vi "SVFA Zoom FFT Spectrum (Mag-Phase).vi"   [LabVIEW 2017]
doc: "Computes the zoom FFT spectrum of <B>scaled signal [EU]</B> and <B>zoom settings</B>. Zoom FFT results are returned in magnitude and phase. Data accumulates each time this VI is called. However, it returns a new spectrum only when sufficient data accumulates. Indicators and subsequent processing should only be called when <B>new spectrum available</B> is TRUE. Wire data to the <B>scaled signal [EU]</B> input to determine the polymorphic instance to use or manually select the instance."
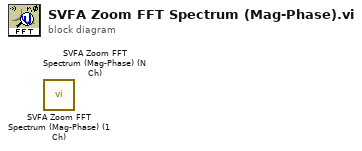
[diagram p0: block diagram]
diagram:
  n1 = call <vilib>:"SVFA Zoom FFT Spectrum (Mag-Phase) (1 Ch).vi"() -> ()  [unwired: 11 in, 9 out]
  n2 = call <vilib>:"SVFA Zoom FFT Spectrum (Mag-Phase) (N Ch).vi"() -> ()  [unwired: 11 in, 9 out]
